vi "Configuration Keys.vi"(8 "error in":errorcluster, 11 "DIG_IO in":refnum<class "DIG_IO.lvclass">) -> (0 "error out":errorcluster, 2 "Required Keys":string[](array[string]), 3 "DIG_IO out":refnum<class "DIG_IO.lvclass">)   [LabVIEW 2019, in "DIG_IO.lvlib" / "DIG_IO.lvclass"]
doc: "Configuration Keys is a dynamic dispatch VI that reads a full inheritance chain's required key list.\n\nThis means each instrument must override this vi, and call the parent method . The end result is a comprehensive list of required keys that must be present in an instrument's config.ini file to correctly function."
uses:
  Library/DIG_IO.lvclass
  Custom Controls/Configuration Keys.ctl
  builds/Instruments/Instruments.lvlibp/Library/Instruments.lvclass
panel:
  in  "Configuration Keys":T1
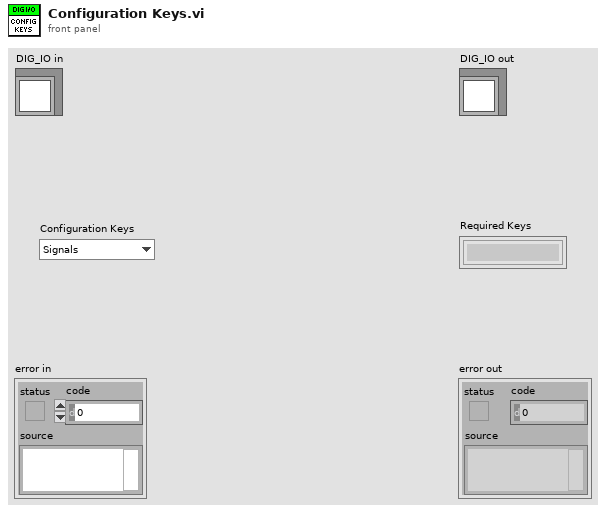
[diagram p1: front panel]
types:
  T1 = typedef "DIG_IO.lvlib/DIG_IO.lvclass/Configuration Keys.ctl" = enum16{"Signals", "CompactLogging"}
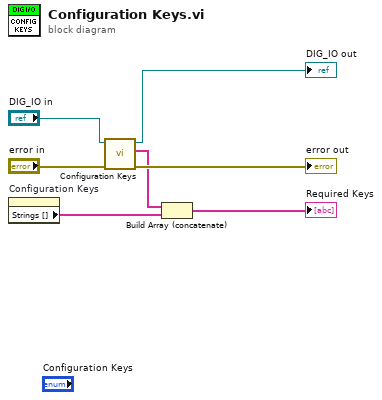
[diagram p0: block diagram]
diagram:
  n1 = property on="Configuration Keys" class="Enum (strict)"() -> ("Strings []"=w2:string[])  [unwired: 2 in, 2 out]
  n2 = call-parent "Configuration Keys.vi"("error in"="error in", "Instruments in"="DIG_IO in") -> ("error out"=→"error out":errorcluster, "Required Keys"=w3:string[], "Instruments out"=→"DIG_IO out":refnum<class "DIG_IO.lvclass">)  [unwired: 7 in]
  n3 = Build Array (concatenate)(w3, w2) -> (→"Required Keys":string[])
